vi "tacometro_xy.vi"(0 "VALOR\nACTUALx":dbl, 5 "MÁXIMO \nVALOR x":dbl, 7 "VALOR\nACTUALy":dbl, 9 "MÁXIMO \nVALORy":dbl) -> (4 "XY Graph":cluster{dbl[], dbl[]}(graph))   [LabVIEW 2023]
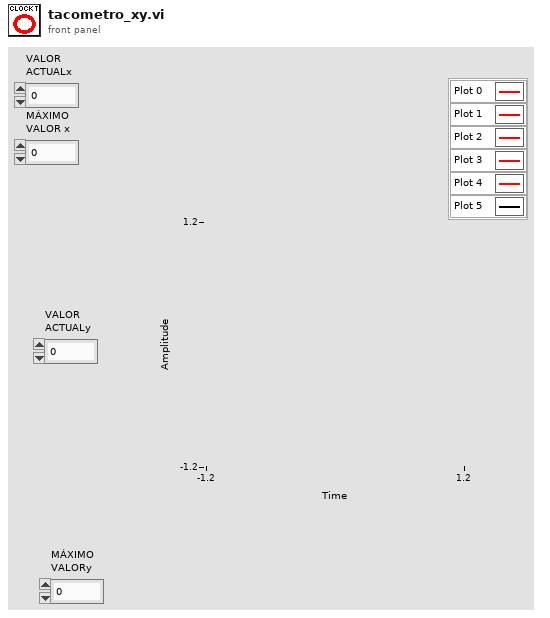
[diagram p1: front panel]
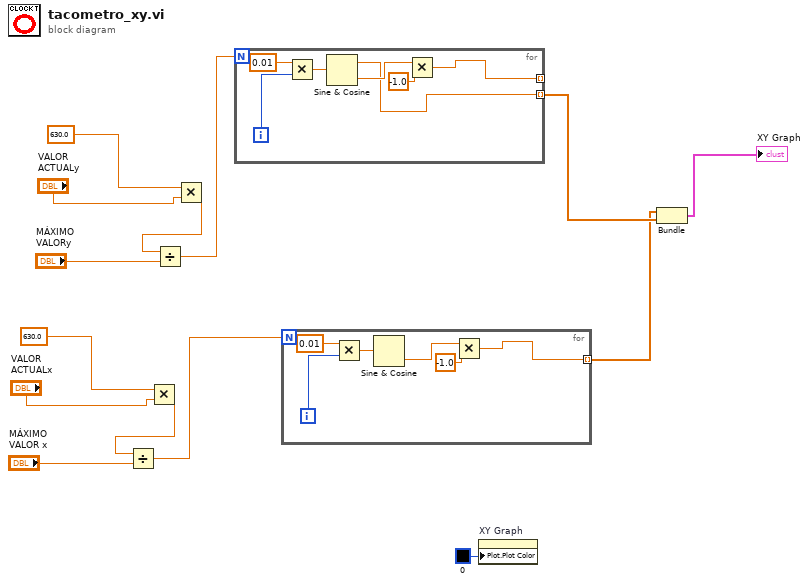
[diagram p0: block diagram]
diagram:
  n1 = Multiply(x=630.0, y="VALOR\nACTUALx") -> (x*y=w4:dbl)
  n2 = Divide(x=w4, y="MÁXIMO \nVALOR x") -> (x/y=w2:dbl)
  n3 = Multiply(x=630.0, y="VALOR\nACTUALy") -> (x*y=w12:dbl)
  n4 = Divide(x=w12, y="MÁXIMO \nVALORy") -> (x/y=w14:dbl)
  n5 = for {
    N: w14 -> [_]
    tunnel: [w15] -> w9 mode=indexing
    tunnel: [w16] -> _ mode=indexing
    i -> [w17]
    n6 = Multiply(x=0.01 ("y"), y=w17) -> (x*y=w19:dbl)
    n7 = Sine & Cosine(0:w19) -> (1:w15:dbl, 2:w20:dbl)
    n8 = Multiply(x=w20, y=-1.0) -> (x*y=w16:dbl)
  }
  n9 = for {
    N: w2 -> [_]
    tunnel: [w22] -> w1 mode=indexing
    i -> [w23]
    n10 = Multiply(x=0.01 ("y"), y=w23) -> (x*y=w25:dbl)
    n11 = Sine & Cosine(0:w25) -> (2:w26:dbl)  [unwired: 1 out]
    n12 = Multiply(x=w26, y=-1.0) -> (x*y=w22:dbl)
  }
  n13 = property on="XY Graph" class="XYGraph (strict)"("Plot.Plot Color"=u32 0) -> ()  [unwired: 2 in, 2 out]
  n14 = Bundle(w1, w9) -> (→"XY Graph":cluster{dbl[], dbl[]})  [unwired: 1 in]
